vi "test_232_imu_MW-AHRSv1_3d.vi"() -> ()   [LabVIEW 2019]
uses:
  Ctrl/cmd_imu.ctl
  <vilib>/picture/3D Picture Control/Object/Create Object (name).vi
  <vilib>/Instr/_visa.llb/VISA Configure Serial Port (Instr).vi
  <vilib>/picture/3D Picture Control/NI_3D Picture Control.lvlib
panel:
  in  "탭 컨트롤":enum32{"3d ui"}(tab)
  out "3D Picture":refnum<vi>(3d-picture)
  out "dir":picture
  out "heading":dbl format="%.1f"
  in  "baud rate":u32=115200 caption="rate"
  in  "Port":refnum<visa-resource-name>="COM24"
  in  "w-data":string="ang"
  out "error out":errorcluster caption="에러 출력"
  in  "w":bool
  out "r buff":u32(graph)
  in  "정지":bool
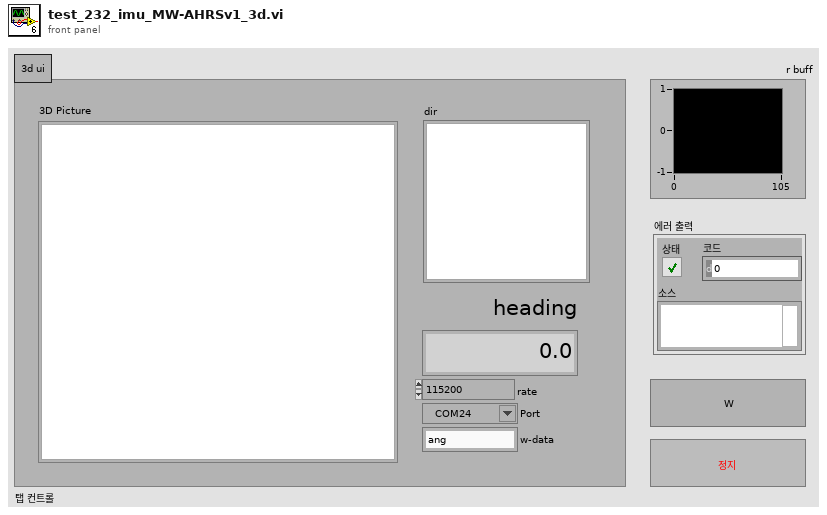
[diagram p1: front panel]
types:
  T1 = typedef "cmd_imu.ctl" = enum16{"ini", "write", "read"}
  T2 = cluster{"angle":dbl[], "acc":dbl[], "mag":dbl[], "gyr":dbl[]}
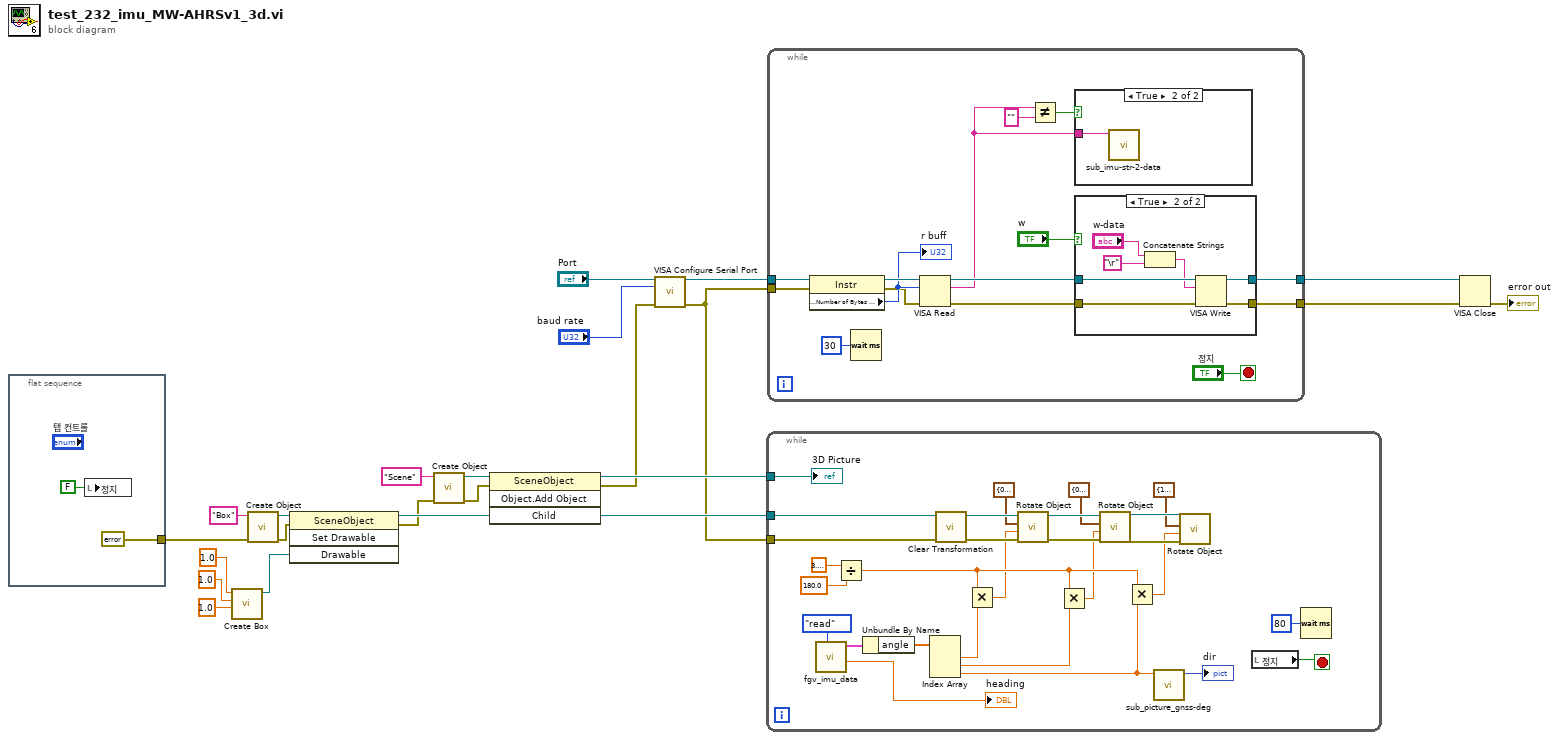
[diagram p0: block diagram]
diagram:
  n1 = flat-sequence {
    tunnel: [errorcluster {"status"=FALSE, "code"=0, "source"=""} ("error in (no error)")] -> w4
    frame #0 {
      n2 = local write "정지"(FALSE ("정지")) -> ()
    }
  }
  n3 = call <vilib>:"Create Box.vi"("Length Z"=sgl 1.0, "Length Y"=sgl 1.0, "Length X"=sgl 1.0) -> ("New Box Refnum"=w13:refnum<vi>)  [unwired: 7 in, 1 out]
  n4 = call-poly <vilib>:"Create Object.vi"("error in (no error)"=w4, "Name"="Box") -> ("error out"=w12:errorcluster, "Scene:New Object"=w11:refnum<vi>)  [unwired: 8 in]
  n5 = invoke class="SceneObject" method="Set Drawable"(reference=w11, error in=w12, "Drawable"=w13) -> (reference out=w17:refnum<vi>, error out=w3:errorcluster)  [unwired: 1 in, 2 out]
  n6 = call-poly <vilib>:"Create Object.vi"("error in (no error)"=w3, "Name"="Scene") -> ("error out"=w16:errorcluster, "Scene:New Object"=w15:refnum<vi>)  [unwired: 8 in]
  n7 = invoke class="SceneObject" method="Object.Add Object"(reference=w15, error in=w16, "Child"=w17) -> (reference out=w6:refnum<vi>, error out=w2:errorcluster, "Child"=w5:refnum<vi>)  [unwired: 1 in, 1 out]
  n8 = call-poly "VISA Configure Serial Port"("VISA resource name"="Port", "baud rate (9600)"="baud rate", "error in (no error)"=w2) -> ("VISA resource name out"=w21:refnum<visa-resource-name>, "error out"=w1:errorcluster)  [unwired: 11 in]
  n9 = while {
    tunnel: w6 -> [w39]
    tunnel: w5 -> [w53]
    tunnel: w1 -> [w30]
    stop <- w36 stop-if-true
    n10 = call "fgv_imu_data.vi"("cmd"=cmd_imu."read") -> ("heading"=→"heading":dbl, "IMD data out"=w34:T2)  [unwired: 7 in, 2 out]
    n11 = Divide(x=3.141592653589793, y=180.0) -> (x/y=w41:dbl)
    n12 = Unbundle By Name(w34) -> ("angle"=w33:dbl[])
    n13 = Index Array(array=w33) -> (element #1=w32:dbl, element #2=w31:dbl, element #3=w28:dbl)  [unwired: 3 in]
    n14 = call <vilib>:"Clear Transformation.vi"("error in (no error)"=w30, "Object Refnum In"=w53) -> ("error out"=w49:errorcluster, "Object Refnum Out"=w50:refnum<vi>)  [unwired: 8 in]
    n15 = Multiply(x=w41, y=w32) -> (x*y=w38:dbl)
    n16 = call <vilib>:"Rotate Object.vi"("error in (no error)"=w49, "Angle"=w38, "Axis"=cluster{"X":sgl, "Y":sgl, "Z":sgl} {"X"=0.0, "Y"=1.0, "Z"=0.0}, "Scene.Object In"=w50) -> ("error out"=w51:errorcluster, "Scene.Object Out"=w52:refnum<vi>)  [unwired: 6 in]
    n17 = Multiply(x=w41, y=w31) -> (x*y=w37:dbl)
    n18 = call <vilib>:"Rotate Object.vi"("error in (no error)"=w51, "Angle"=w37, "Axis"=cluster{"X":sgl, "Y":sgl, "Z":sgl} {"X"=0.0, "Y"=0.0, "Z"=1.0}, "Scene.Object In"=w52) -> ("error out"=w44:errorcluster, "Scene.Object Out"=w45:refnum<vi>)  [unwired: 6 in]
    n19 = Multiply(x=w41, y=w28) -> (x*y=w40:dbl)
    n20 = call "sub_picture_gnss-deg.vi"("deg_gps"=w28) -> ("new picture"=→"dir":picture)  [unwired: 10 in]
    n21 = call <vilib>:"Rotate Object.vi"("error in (no error)"=w44, "Angle"=w40, "Axis"=cluster{"X":sgl, "Y":sgl, "Z":sgl} {"X"=1.0, "Y"=0.0, "Z"=0.0}, "Scene.Object In"=w45) -> ()  [unwired: 6 in, 2 out]
    n22 = local read "정지"() -> (w36:bool)
    n23 = Wait (ms)(milliseconds to wait=u32 80 ("대기 시간 (ms)")) -> ()  [unwired: 1 out]
    "3D Picture" <- w39
  }
  n24 = while {
    tunnel: w1 -> [w63]
    tunnel: w21 -> [w62]
    tunnel: [w58] -> w19
    tunnel: [w57] -> w18
    stop <- "정지" stop-if-true
    n25 = property class="Instr"(reference=w62, error in=w63) -> (reference out=w67:refnum<visa-resource-name>, error out=w64:errorcluster, "Serial Settings:Number of Bytes at Serial Port"=w65:u32)
    "r buff" <- w65
    n26 = Wait (ms)(milliseconds to wait=u32 30 ("대기 시간 (ms)")) -> ()  [unwired: 1 out]
    n27 = VISA Read(VISA resource name=w67, byte count=w65, error in (no error)=w64) -> (VISA resource name out=w59:refnum<visa-resource-name>, read buffer=w54:string, error out=w60:errorcluster)  [unwired: 1 out]
    n28 = Not Equal?(x=w54, y="") -> (x != y?=w56:bool)
    n29 = case shown="True" w56 {
      tunnel: w54 -> [_ w69]
      frame False {
      }
      frame True {
        n30 = call "sub_imu-str-2-data.vi"("read buffer"=w69) -> ()  [unwired: 9 in, 2 out]
      }
    }
    n31 = case shown="True" "w" {
      tunnel: w59 -> [w71 w78]
      tunnel: [w71 w77] -> w58
      tunnel: w60 -> [w70 w76]
      tunnel: [w70 w75] -> w57
      frame False {
      }
      frame True {
        n32 = Concatenate Strings("w-data", "\r") -> (w72:string)
        n33 = VISA Write(VISA resource name=w78, write buffer=w72, error in (no error)=w76) -> (VISA resource name out=w77:refnum<visa-resource-name>, error out=w75:errorcluster)  [unwired: 1 out]
      }
    }
  }
  n34 = VISA Close(VISA resource name=w19, error in (no error)=w18) -> (error out=→"error out":errorcluster)
